vi "HID - FPGA VI.vi"() -> ()   [LabVIEW 2015]
uses:
  <vilib>/rvi/DataTransferAndStorage/Container/XNode/niFpgaContainer.xnode
  <vilib>/eio/EIONode/EIONode.xnode
  <vilib>/rvi/eio/common/nirviEmuTemplateMethod_errors.vi
  <vilib>/rvi/Memory/Memory_Emulation/nirvimemoryFastEmulation.vi
  <vilib>/rvi/Memory/Memory_Emulation/nirvimemoryEmulation.vi
  <vilib>/rvi/interface/RandomDataEmulation/nirviRandomDataFpgaReadWriteTemplate.vi
  <vilib>/rvi/FIFO/Fifo_Resource/niFpgaFifoEmulationRefIn.vi
panel:
  in  "Memory write timer (uSec)":u8=20
  in  "Count(mSec)":u16 caption="FIFO Consumer Loop Timer(mSec)"
  in  "Row timer":u32 caption="Row Timer(uSec)"
  in  "Color Background":T1(ring)
  in  "Color":T1(ring)
  in  "Line Shift?":bool
  in  "Write State":enum16{"Running", "Off"}(ring)
  # "Loop Timing Controls"
  # "Color Options"
  # "Other Options"
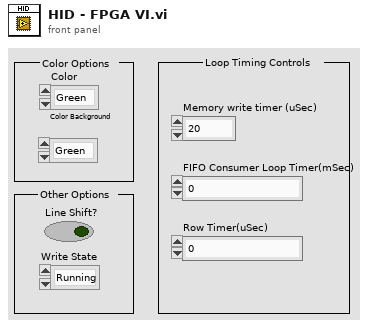
[diagram p1: front panel]
types:
  T1 = enum16{"Green", "Blue", "Red", "White", "Pink", "Yellow", "Turquoise", "Black"}
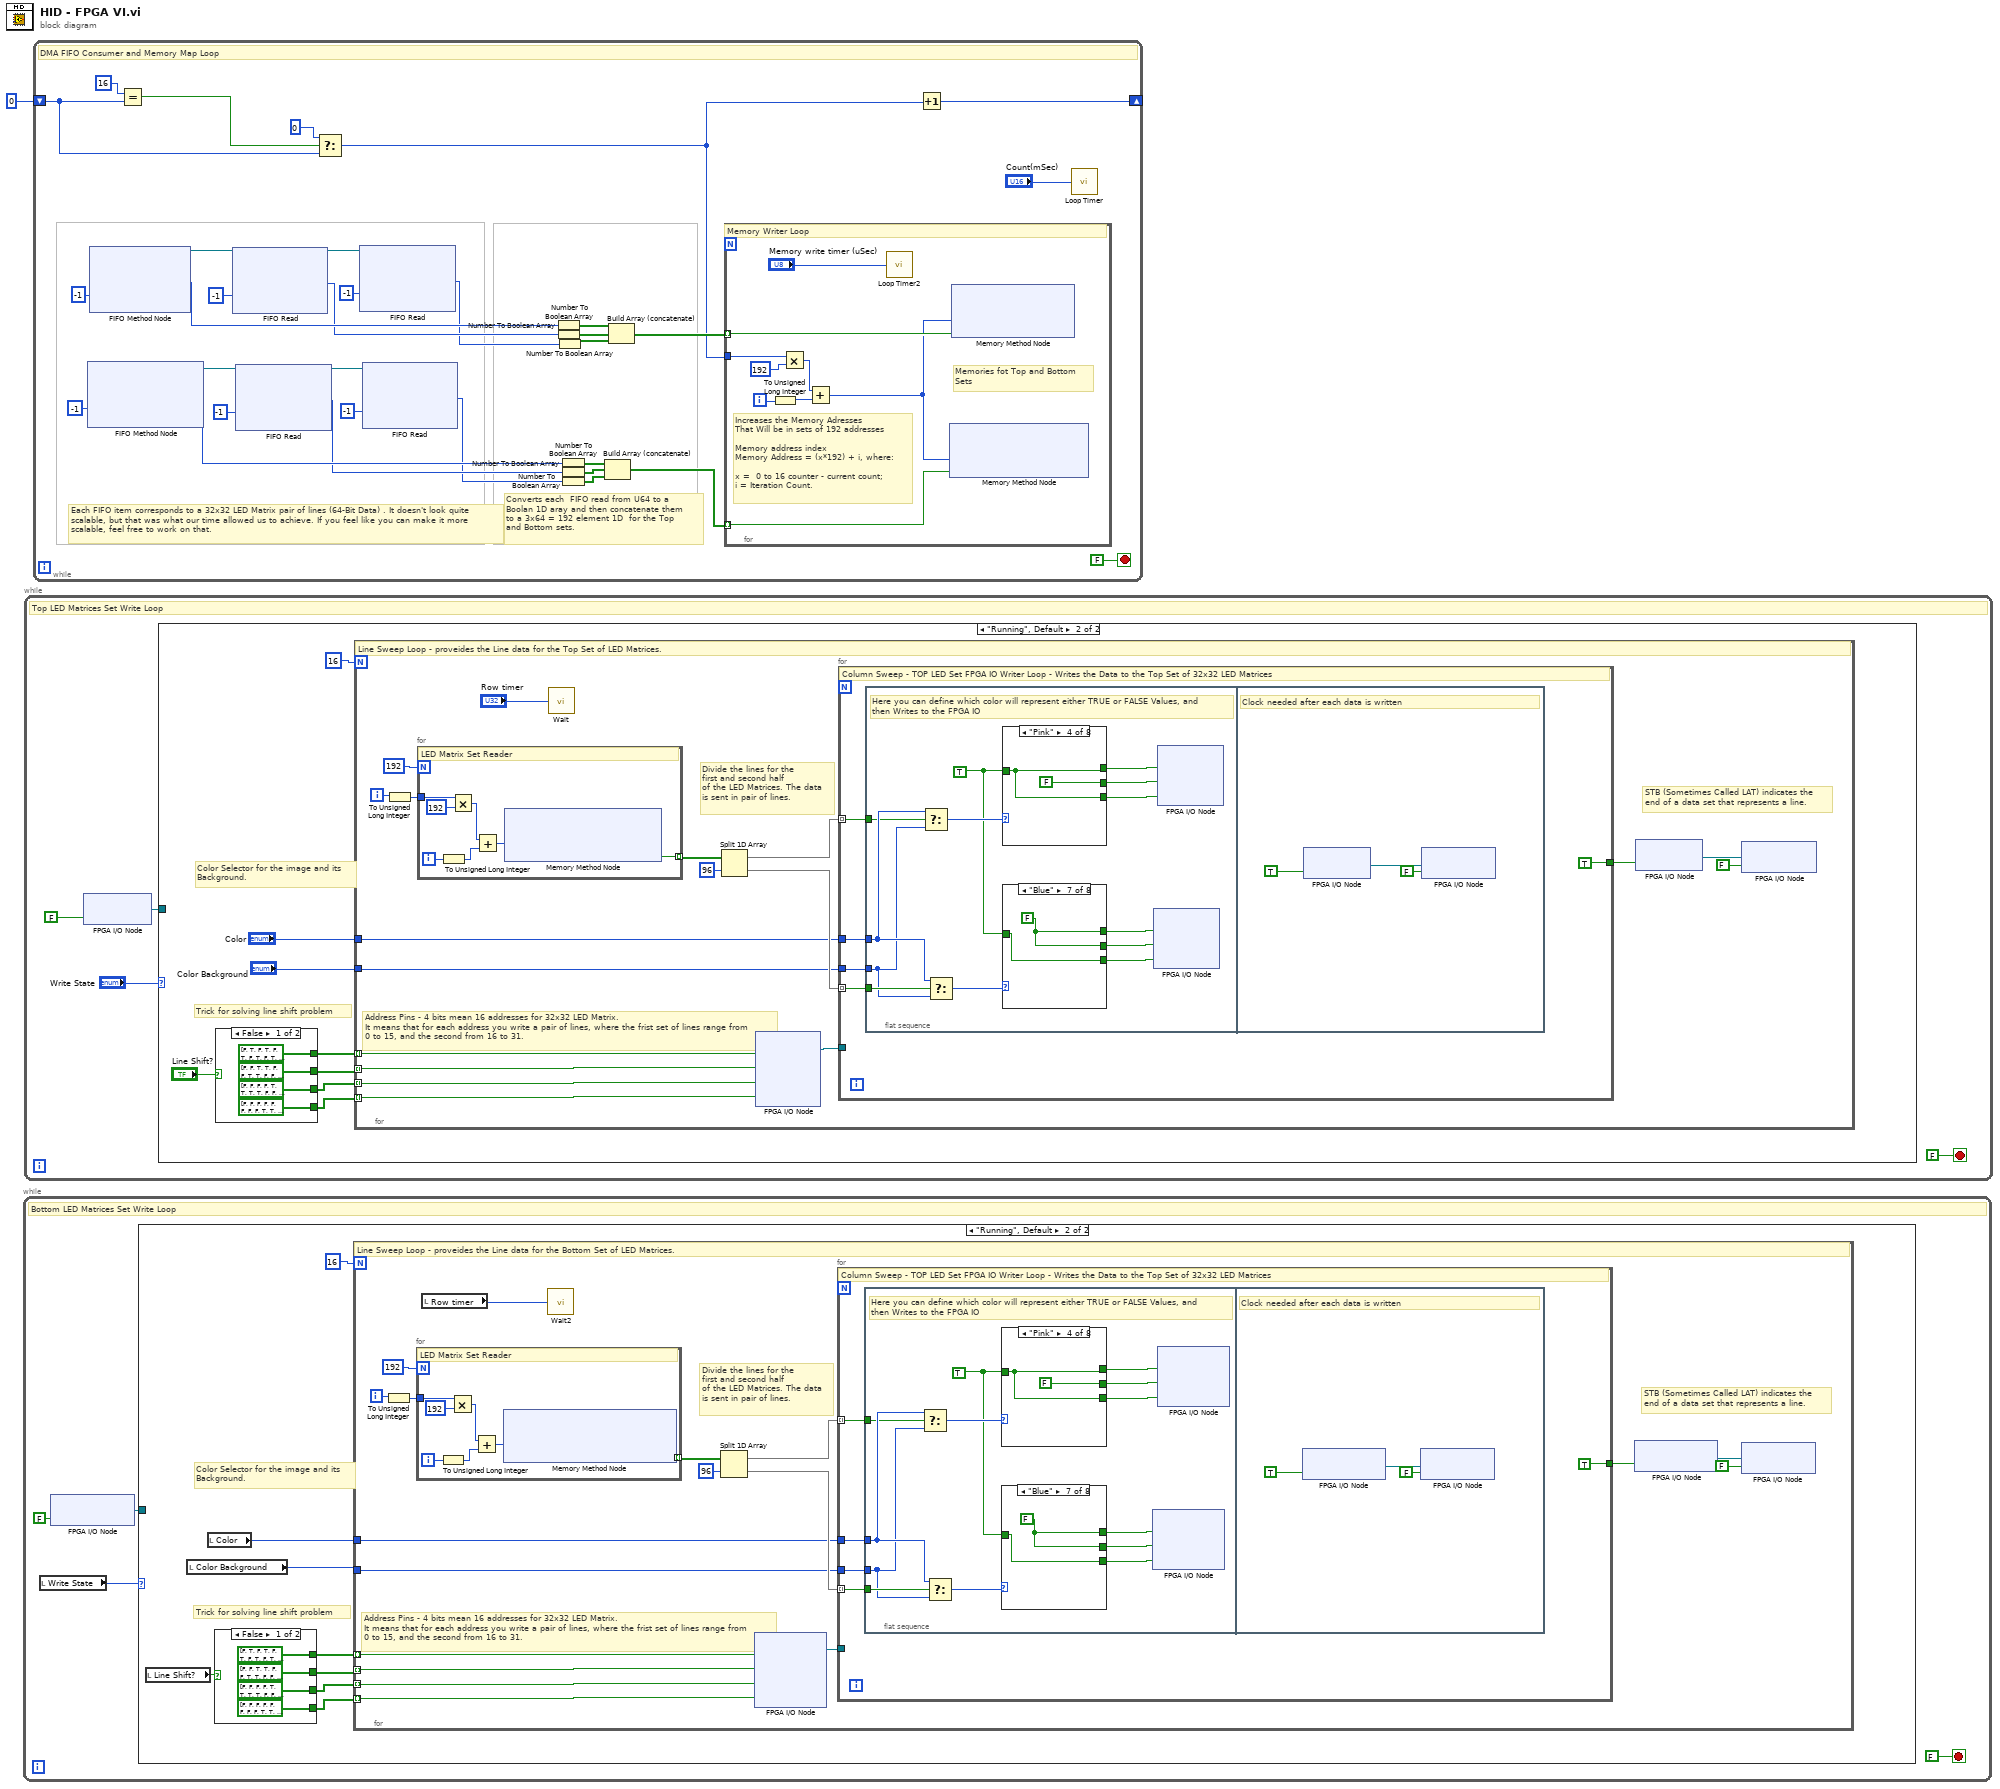
[diagram p0: block diagram]
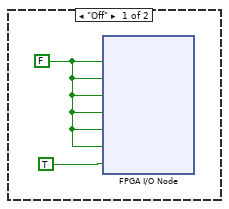
[diagram p2: hidden frame]
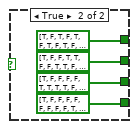
[diagram p3: hidden frame]
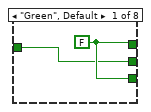
[diagram p4: hidden frame]
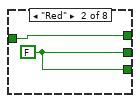
[diagram p5: hidden frame]
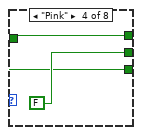
[diagram p7: hidden frame]
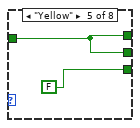
[diagram p8: hidden frame]
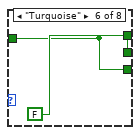
[diagram p9: hidden frame]
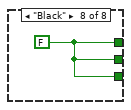
[diagram p10: hidden frame]
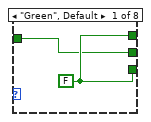
[diagram p11: hidden frame]
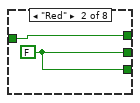
[diagram p12: hidden frame]
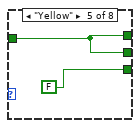
[diagram p14: hidden frame]
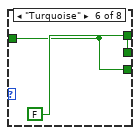
[diagram p15: hidden frame]
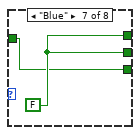
[diagram p16: hidden frame]
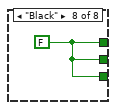
[diagram p17: hidden frame]
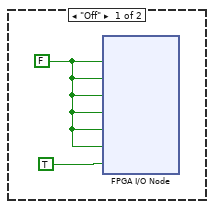
[diagram p18: hidden frame]
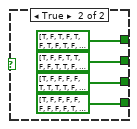
[diagram p19: hidden frame]
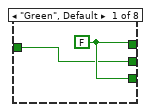
[diagram p20: hidden frame]
diagram:
  n1 = while {
    stop <- FALSE stop-if-true
    # "Bottom LED Matrices Set Write Loop"
    n2 = local read "Write State"() -> (w2:enum16{"Running", "Off"})
    n3 = xnode "FPGA I/O Node"("Bot13 CLK"=FALSE ("13 CLK 3")) -> ("FPGA I/O Out"=w3:refnum<k21>)  [unwired: 1 in]
    n4 = case shown="\"Running\", Default" w2 {
      tunnel: w3 -> [_ _]
      frame "Off" {
        w7 = FALSE ("1 R0")
        n5 = xnode "FPGA I/O Node"("Bot1 R0"=w7, "Bot2 G0"=w7, "Bot3 B0"=w7, "Bot5 R1"=w7, "Bot6 G1"=w7, "Bot7 B1"=w7, "Bot15 OE"=TRUE ("15 OE")) -> ()  [unwired: 7 in, 7 out]
      }
      frame "Running", Default {
        # "Trick for solving line shift problem"
        # "Color Selector for the image and its\nBackground."
        n6 = local read "Line Shift?"() -> (w8:bool)
        n7 = local read "Color Background"() -> (w9:T1)
        n8 = local read "Color"() -> (w10:T1)
        n9 = case shown="False" w8 {
          tunnel: [bool[] [FALSE, TRUE, FALSE, TRUE, FALSE, TRUE, FALSE, TRUE, FALSE, TRUE, FALSE, TRUE, FALSE, TRUE, FALSE, TRUE] ("Logic A") bool[] [TRUE, FALSE, TRUE, FALSE, TRUE, FALSE, TRUE, FALSE, TRUE, FALSE, TRUE, FALSE, TRUE, FALSE, TRUE, FALSE] ("Logic A")] -> w14
          tunnel: [bool[] [FALSE, FALSE, TRUE, TRUE, FALSE, FALSE, TRUE, TRUE, FALSE, FALSE, TRUE, TRUE, FALSE, FALSE, TRUE, TRUE] ("Logic B") bool[] [TRUE, FALSE, FALSE, TRUE, TRUE, FALSE, FALSE, TRUE, TRUE, FALSE, FALSE, TRUE, TRUE, FALSE, FALSE, TRUE] ("Logic B")] -> w13
          tunnel: [bool[] [FALSE, FALSE, FALSE, FALSE, TRUE, TRUE, TRUE, TRUE, FALSE, FALSE, FALSE, FALSE, TRUE, TRUE, TRUE, TRUE] ("Logic C") bool[] [TRUE, FALSE, FALSE, FALSE, FALSE, TRUE, TRUE, TRUE, TRUE, FALSE, FALSE, FALSE, FALSE, TRUE, TRUE, TRUE] ("Logic C")] -> w12
          tunnel: [bool[] [FALSE, FALSE, FALSE, FALSE, FALSE, FALSE, FALSE, FALSE, TRUE, TRUE, TRUE, TRUE, TRUE, TRUE, TRUE, TRUE] ("Logic D") bool[] [TRUE, FALSE, FALSE, FALSE, FALSE, FALSE, FALSE, FALSE, FALSE, TRUE, TRUE, TRUE, TRUE, TRUE, TRUE, TRUE] ("Logic D")] -> w11
          frame False {
          }
          frame True {
          }
        }
        n10 = for {
          N: 16 -> [_]
          tunnel: w14 -> [w29] mode=indexing
          tunnel: w13 -> [w28] mode=indexing
          tunnel: w12 -> [w27] mode=indexing
          tunnel: w11 -> [w26] mode=indexing
          tunnel: w10 -> [w37]
          tunnel: w9 -> [w25]
          i -> [w39]
          # "Address Pins - 4 bits mean 16 addresses for 32x32 LED Matrix.\nIt means that for each address you write a pair of lines, where the frist set of lines range from\n0 to 15, and the second from 16 to 31."
          # "STB (Sometimes Called LAT) indicates the\nend of a data set that represents a line."
          # "Divide the lines for the\nfirst and second half\nof the LED Matrices. The data\nis sent in pair of lines."
          # "Line Sweep Loop - proveides the Line data for the Bottom Set of LED Matrices."
          n11 = To Unsigned Long Integer(number=w39) -> (unsigned 32bit integer=w35:u32)
          n12 = for {
            N: 192 -> [_]
            tunnel: w35 -> [w46]
            tunnel: [w43] -> w36 mode=indexing
            i -> [w45]
            # "LED Matrix Set Reader"
            n13 = To Unsigned Long Integer(number=w45) -> (unsigned 32bit integer=w44:u32)
            n14 = Multiply(x=w46, y=u32 192) -> (x*y=w47:u32)
            n15 = Add(x=w47, y=w44) -> (x+y=w42:u32)
            n16 = xnode ("Memory Method Node")("Address"=w42) -> ("Data"=w43:bool)  [unwired: 1 in, 1 out]
          }
          n17 = local read "Row timer"() -> (w24:u32)
          n18 = call "Wait2"("Count(uSec)"=w24) -> ()  [unwired: 1 out]
          n19 = Split 1D Array(array=w36, index=96) -> (first subarray=w34:bool[], second subarray=w40:bool[])
          n20 = xnode "FPGA I/O Node"("Bot9 A"=w29, "Bot10 B"=w28, "Bot11 C"=w27, "Bot12 D"=w26) -> ("FPGA I/O Out"=w30:refnum<k21>)  [unwired: 4 in, 3 out]
          n21 = for {
            tunnel: w34 -> [w53] mode=indexing
            tunnel: w40 -> [w52] mode=indexing
            tunnel: w37 -> [w51]
            tunnel: [TRUE ("14 STB")] -> w33
            tunnel: w30 -> [_]
            tunnel: w25 -> [w49]
            # "Column Sweep - TOP LED Set FPGA IO Writer Loop - Writes the Data to the Top Set of 32x32 LED Matrices"
            n22 = flat-sequence {
              tunnel: w53 -> [w55]
              tunnel: w52 -> [w59]
              tunnel: w51 -> [w58]
              tunnel: w49 -> [w57]
              frame #0 {
                w54 = TRUE
                # "Here you can define which color will represent either TRUE or FALSE Values, and \nthen Writes to the FPGA IO"
                n23 = Select(t=w58, s=w55, f=w57) -> (s? t:f=w60:T1)
                n24 = Select(t=w58, s=w59, f=w57) -> (s? t:f=w56:T1)
                n25 = case shown="\"Pink\"" w60 {
                  tunnel: [w82 w83 w85 w86 w88 FALSE ("1 R0") w93 w94] -> w66
                  tunnel: [w81 w84 w85 FALSE ("1 R0") w88 w90 w93 w94] -> w65
                  tunnel: [w82 w84 w85 w86 FALSE ("1 R0") w90 w92 w94] -> w64
                  tunnel: w54 -> [w81 w83 w85 w86 w88 w90 w92 _]
                  frame "Green", Default {
                    w82 = FALSE ("1 R0")
                  }
                  frame "Red" {
                    w84 = FALSE ("1 R0")
                  }
                  frame "White" {
                  }
                  frame "Pink" {
                  }
                  frame "Yellow" {
                  }
                  frame "Turquoise" {
                  }
                  frame "Blue" {
                    w93 = FALSE ("1 R0")
                  }
                  frame "Black" {
                    w94 = FALSE
                  }
                }
                n26 = case shown="\"Blue\"" w56 {
                  tunnel: [w68 w69 w71 w72 w74 FALSE ("1 R0") w79 w80] -> w63
                  tunnel: [w67 w70 w71 FALSE ("1 R0") w74 w76 w79 w80] -> w62
                  tunnel: [w68 w70 w71 w72 FALSE ("1 R0") w76 w78 w80] -> w61
                  tunnel: w54 -> [w67 w69 w71 w72 w74 w76 w78 _]
                  frame "Green", Default {
                    w68 = FALSE ("1 R0")
                  }
                  frame "Red" {
                    w70 = FALSE ("1 R0")
                  }
                  frame "White" {
                  }
                  frame "Pink" {
                  }
                  frame "Yellow" {
                  }
                  frame "Turquoise" {
                  }
                  frame "Blue" {
                    w79 = FALSE ("1 R0")
                  }
                  frame "Black" {
                    w80 = FALSE
                  }
                }
                n27 = xnode "FPGA I/O Node"("Bot5 R1"=w63, "Bot6 G1"=w62, "Bot7 B1"=w61) -> ()  [unwired: 3 in, 3 out]
                n28 = xnode "FPGA I/O Node"("Bot1 R0"=w66, "Bot2 G0"=w65, "Bot3 B0"=w64) -> ()  [unwired: 3 in, 3 out]
              }
              frame #1 {
                # "Clock needed after each data is written"
                n29 = xnode "FPGA I/O Node"("Bot13 CLK"=TRUE ("13 CLK 3")) -> ("FPGA I/O Out"=w95:refnum<k21>)  [unwired: 1 in]
                n30 = xnode "FPGA I/O Node"("I/O Item"=FALSE, "FPGA I/O In"=w95) -> ()  [unwired: 1 out]
              }
            }
          }
          n31 = xnode "FPGA I/O Node"("Bot14 STB"=w33) -> ("FPGA I/O Out"=w31:refnum<k21>)  [unwired: 1 in]
          n32 = xnode "FPGA I/O Node"("I/O Item"=FALSE ("14 STB"), "FPGA I/O In"=w31) -> ()  [unwired: 1 out]
        }
      }
    }
  }
  n33 = while {
    stop <- FALSE stop-if-true
    # "Top LED Matrices Set Write Loop"
    n34 = xnode "FPGA I/O Node"("13 CLK"=FALSE ("13 CLK 3")) -> ("FPGA I/O Out"=w98:refnum<k21>)  [unwired: 1 in]
    n35 = case shown="\"Running\", Default" "Write State" {
      tunnel: w98 -> [_ _]
      frame "Off" {
        w103 = FALSE ("1 R0")
        n36 = xnode "FPGA I/O Node"("1 R0"=w103, "2 G0"=w103, "3 B0"=w103, "5 R1"=w103, "6 G1"=w103, "7 B1"=w103, "15 OE"=TRUE) -> ()  [unwired: 7 in, 7 out]
      }
      frame "Running", Default {
        # "Trick for solving line shift problem"
        # "Color Selector for the image and its\nBackground."
        n37 = case shown="False" "Line Shift?" {
          tunnel: [bool[] [FALSE, TRUE, FALSE, TRUE, FALSE, TRUE, FALSE, TRUE, FALSE, TRUE, FALSE, TRUE, FALSE, TRUE, FALSE, TRUE] ("Logic A") bool[] [TRUE, FALSE, TRUE, FALSE, TRUE, FALSE, TRUE, FALSE, TRUE, FALSE, TRUE, FALSE, TRUE, FALSE, TRUE, FALSE] ("Logic A")] -> w109
          tunnel: [bool[] [FALSE, FALSE, TRUE, TRUE, FALSE, FALSE, TRUE, TRUE, FALSE, FALSE, TRUE, TRUE, FALSE, FALSE, TRUE, TRUE] ("Logic B") bool[] [TRUE, FALSE, FALSE, TRUE, TRUE, FALSE, FALSE, TRUE, TRUE, FALSE, FALSE, TRUE, TRUE, FALSE, FALSE, TRUE] ("Logic B")] -> w108
          tunnel: [bool[] [FALSE, FALSE, FALSE, FALSE, TRUE, TRUE, TRUE, TRUE, FALSE, FALSE, FALSE, FALSE, TRUE, TRUE, TRUE, TRUE] ("Logic C") bool[] [TRUE, FALSE, FALSE, FALSE, FALSE, TRUE, TRUE, TRUE, TRUE, FALSE, FALSE, FALSE, FALSE, TRUE, TRUE, TRUE] ("Logic C")] -> w107
          tunnel: [bool[] [FALSE, FALSE, FALSE, FALSE, FALSE, FALSE, FALSE, FALSE, TRUE, TRUE, TRUE, TRUE, TRUE, TRUE, TRUE, TRUE] ("Logic D") bool[] [TRUE, FALSE, FALSE, FALSE, FALSE, FALSE, FALSE, FALSE, FALSE, TRUE, TRUE, TRUE, TRUE, TRUE, TRUE, TRUE] ("Logic D")] -> w106
          frame False {
          }
          frame True {
          }
        }
        n38 = for {
          N: 16 -> [_]
          tunnel: w109 -> [w124] mode=indexing
          tunnel: w108 -> [w123] mode=indexing
          tunnel: w107 -> [w122] mode=indexing
          tunnel: w106 -> [w121] mode=indexing
          tunnel: "Color" -> [w132]
          tunnel: "Color Background" -> [w120]
          i -> [w135]
          # "Address Pins - 4 bits mean 16 addresses for 32x32 LED Matrix.\nIt means that for each address you write a pair of lines, where the frist set of lines range from\n0 to 15, and the second from 16 to 31."
          # "STB (Sometimes Called LAT) indicates the\nend of a data set that represents a line."
          # "Divide the lines for the\nfirst and second half\nof the LED Matrices. The data\nis sent in pair of lines."
          # "Line Sweep Loop - proveides the Line data for the Top Set of LED Matrices."
          n39 = To Unsigned Long Integer(number=w135) -> (unsigned 32bit integer=w130:u32)
          n40 = for {
            N: 192 -> [_]
            tunnel: w130 -> [w142]
            tunnel: [w139] -> w131 mode=indexing
            i -> [w141]
            # "LED Matrix Set Reader"
            n41 = To Unsigned Long Integer(number=w141) -> (unsigned 32bit integer=w140:u32)
            n42 = Multiply(x=w142, y=u32 192) -> (x*y=w143:u32)
            n43 = Add(x=w143, y=w140) -> (x+y=w138:u32)
            n44 = xnode ("Memory Method Node")("Address"=w138) -> ("Data"=w139:bool)  [unwired: 1 in, 1 out]
          }
          n45 = call "Wait"("Count(uSec)"="Row timer") -> ()  [unwired: 1 out]
          n46 = Split 1D Array(array=w131, index=96) -> (first subarray=w129:bool[], second subarray=w136:bool[])
          n47 = xnode "FPGA I/O Node"("9 A"=w124, "10 B"=w123, "11 C"=w122, "12 D"=w121) -> ("FPGA I/O Out"=w125:refnum<k21>)  [unwired: 4 in, 3 out]
          n48 = for {
            tunnel: w129 -> [w149] mode=indexing
            tunnel: w136 -> [w148] mode=indexing
            tunnel: w132 -> [w147]
            tunnel: [TRUE ("14 STB")] -> w128
            tunnel: w125 -> [_]
            tunnel: w120 -> [w145]
            # "Column Sweep - TOP LED Set FPGA IO Writer Loop - Writes the Data to the Top Set of 32x32 LED Matrices"
            n49 = flat-sequence {
              tunnel: w149 -> [w151]
              tunnel: w148 -> [w155]
              tunnel: w147 -> [w154]
              tunnel: w145 -> [w153]
              frame #0 {
                w150 = TRUE
                # "Here you can define which color will represent either TRUE or FALSE Values, and \nthen Writes to the FPGA IO"
                n50 = Select(t=w154, s=w151, f=w153) -> (s? t:f=w156:T1)
                n51 = Select(t=w154, s=w155, f=w153) -> (s? t:f=w152:T1)
                n52 = case shown="\"Pink\"" w156 {
                  tunnel: [w178 w179 w181 w182 w184 FALSE ("1 R0") w189 w190] -> w162
                  tunnel: [w177 w180 w181 FALSE ("1 R0") w184 w186 w189 w190] -> w161
                  tunnel: [w178 w180 w181 w182 FALSE ("1 R0") w186 w188 w190] -> w160
                  tunnel: w150 -> [w177 w179 w181 w182 w184 w186 w188 _]
                  frame "Green", Default {
                    w178 = FALSE ("1 R0")
                  }
                  frame "Red" {
                    w180 = FALSE ("1 R0")
                  }
                  frame "White" {
                  }
                  frame "Pink" {
                  }
                  frame "Yellow" {
                  }
                  frame "Turquoise" {
                  }
                  frame "Blue" {
                    w189 = FALSE ("1 R0")
                  }
                  frame "Black" {
                    w190 = FALSE
                  }
                }
                n53 = case shown="\"Blue\"" w152 {
                  tunnel: [w164 w165 w167 w168 w170 FALSE ("1 R0") w175 w176] -> w159
                  tunnel: [w163 w166 w167 FALSE ("1 R0") w170 w172 w175 w176] -> w158
                  tunnel: [w164 w166 w167 w168 FALSE ("1 R0") w172 w174 w176] -> w157
                  tunnel: w150 -> [w163 w165 w167 w168 w170 w172 w174 _]
                  frame "Green", Default {
                    w164 = FALSE ("1 R0")
                  }
                  frame "Red" {
                    w166 = FALSE ("1 R0")
                  }
                  frame "White" {
                  }
                  frame "Pink" {
                  }
                  frame "Yellow" {
                  }
                  frame "Turquoise" {
                  }
                  frame "Blue" {
                    w175 = FALSE ("1 R0")
                  }
                  frame "Black" {
                    w176 = FALSE
                  }
                }
                n54 = xnode "FPGA I/O Node"("5 R1"=w159, "6 G1"=w158, "7 B1"=w157) -> ()  [unwired: 3 in, 3 out]
                n55 = xnode "FPGA I/O Node"("1 R0"=w162, "2 G0"=w161, "3 B0"=w160) -> ()  [unwired: 3 in, 3 out]
              }
              frame #1 {
                # "Clock needed after each data is written"
                n56 = xnode "FPGA I/O Node"("13 CLK"=TRUE ("13 CLK 3")) -> ("FPGA I/O Out"=w191:refnum<k21>)  [unwired: 1 in]
                n57 = xnode "FPGA I/O Node"("I/O Item"=FALSE, "FPGA I/O In"=w191) -> ()  [unwired: 1 out]
              }
            }
          }
          n58 = xnode "FPGA I/O Node"("14 STB"=w128) -> ("FPGA I/O Out"=w126:refnum<k21>)  [unwired: 1 in]
          n59 = xnode "FPGA I/O Node"("I/O Item"=FALSE ("14 STB"), "FPGA I/O In"=w126) -> ()  [unwired: 1 out]
        }
      }
    }
  }
  n60 = while {
    shift-right: [w224] -> _
    shift-left: u32 0 -> [w195]
    stop <- FALSE stop-if-true
    # "Converts each  FIFO read from U64 to a \nBoolan 1D aray and then concatenate them \nto a 3x64 = 192 element 1D  for the Top \nand Bottom sets."
    # "Each FIFO item corresponds to a 32x32 LED Matrix pair of lines (64-Bit Data) . It doesn't look quite\nscalable, but that was what our time allowed us to achieve. If you feel like you can make it more \nscalable, feel free to work on that."
    # "DMA FIFO Consumer and Memory Map Loop"
    n61 = xnode ("FIFO Method Node")("Timeout"=-1) -> ("Element"=w219:u64, "FIFO Out"=w210:refnum<k21>)  [unwired: 1 in, 1 out]
    n62 = xnode ("FIFO Method Node")("Timeout"=-1) -> ("Element"=w222:u64, "FIFO Out"=w215:refnum<k21>)  [unwired: 1 in, 1 out]
    n63 = Equal?(x=u32 16, y=w195) -> (x = y?=w198:bool)
    n64 = xnode ("FIFO Read")("Timeout"=-1, "FIFO In"=w215) -> ("Element"=w221:u64, "FIFO Out"=w213:refnum<k21>)  [unwired: 1 out]
    n65 = xnode ("FIFO Read")("Timeout"=-1, "FIFO In"=w210) -> ("Element"=w218:u64, "FIFO Out"=w209:refnum<k21>)  [unwired: 1 out]
    n66 = Select(t=u32 0, s=w198, f=w195) -> (s? t:f=w194:u32)
    n67 = xnode ("FIFO Read")("Timeout"=-1, "FIFO In"=w213) -> ("Element"=w220:u64)  [unwired: 2 out]
    n68 = xnode ("FIFO Read")("Timeout"=-1, "FIFO In"=w209) -> ("Element"=w217:u64)  [unwired: 2 out]
    n69 = Number To Boolean Array(number=w222) -> (Boolean array=w203:bool[])
    n70 = Number To Boolean Array(number=w221) -> (Boolean array=w202:bool[])
    n71 = Number To Boolean Array(number=w220) -> (Boolean array=w201:bool[])
    n72 = Number To Boolean Array(number=w219) -> (Boolean array=w206:bool[])
    n73 = Number To Boolean Array(number=w218) -> (Boolean array=w204:bool[])
    n74 = Number To Boolean Array(number=w217) -> (Boolean array=w205:bool[])
    n75 = Build Array (concatenate)(w206, w204, w205) -> (w223:bool[])
    n76 = Build Array (concatenate)(w203, w202, w201) -> (w199:bool[])
    n77 = for {
      tunnel: w194 -> [w227]
      tunnel: w199 -> [w229] mode=indexing
      tunnel: w223 -> [w228] mode=indexing
      i -> [w232]
      # "Memories fot Top and Bottom\nSets"
      # "Increases the Memory Adresses\nThat Will be in sets of 192 addresses\n\nMemory address index\nMemory Address = (x*192) + i, where:\n\nx =  0 to 16 counter - current count;\ni = Iteration Count."
      # "Memory Writer Loop"
      n78 = To Unsigned Long Integer(number=w232) -> (unsigned 32bit integer=w231:u32)
      n79 = Multiply(x=w227, y=u32 192) -> (x*y=w233:u32)
      n80 = Add(x=w233, y=w231) -> (x+y=w226:u32)
      n81 = call "Loop Timer2"("Count(uSec)"="Memory write timer (uSec)") -> ()  [unwired: 1 out]
      n82 = xnode ("Memory Method Node")("Address"=w226, "Data"=w228) -> ()  [unwired: 1 in, 1 out]
      n83 = xnode ("Memory Method Node")("Address"=w226, "Data"=w229) -> ()  [unwired: 1 in, 1 out]
    }
    n84 = Increment(x=w194) -> (x+1=w224:u32)
    n85 = call "Loop Timer"("Count(mSec)"="Count(mSec)") -> ()  [unwired: 1 out]
  }
